vi "memory_load_C_1.vi"() -> (0 "Init Data Out":fxp<+/-,32,16>[][](array[numeric]))   [LabVIEW 2020]
panel:
  out "size(s)":i32[](array[numeric])
  # "For Initialization VI requirements and help, please read directions located on Block Diagram."
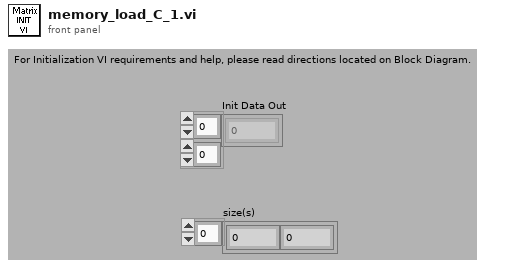
[diagram p1: front panel]
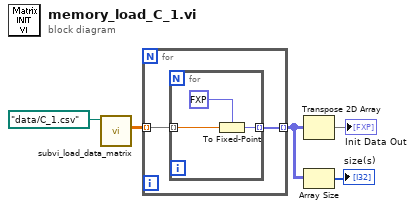
[diagram p0: block diagram]
diagram:
  n1 = call "subvi_load_data_matrix.vi"("default name"=path "data/C_1.csv") -> ("array"=w3:dbl[][])  [unwired: 10 in]
  n2 = for {
    tunnel: w3 -> [w7] mode=indexing
    tunnel: [w6] -> w2 mode=indexing
    n3 = for {
      tunnel: w7 -> [w10] mode=indexing
      tunnel: [w9] -> w6 mode=indexing
      n4 = To Fixed-Point(fixed-point type=fxp<+/-,32,16> 0.0 ("fixed-point"), number=w10) -> (fixed-point=w9:fxp<+/-,32,16>)
    }
  }
  n5 = Transpose 2D Array(2D array=w2) -> (transposed array=→"Init Data Out":fxp<+/-,32,16>[][])
  n6 = Array Size(array=w2) -> (size(s)=→"size(s)":i32[])
